vi "Create Precise Ramp Int16.vi"(8 "error in (no error)":errorcluster, 10 "Waveform":T1={"Start"=1.0, "End"=256.0, "Time"=1.0} {"Start" min=0.0 max=1.0 format="%.2f"; "Time" min=0.0 max=1.0 format="%.2f"}) -> (0 "error out":errorcluster, 2 "Waveform Data":dbl[](array[numeric]))   [LabVIEW 2013]
uses:
  PreciseRampWaveform.ctl
  <vilib>/Analysis/1siggen.llb/Ramp Pattern by Samples.vi
  <vilib>/Analysis/NI_AALBase.lvlib
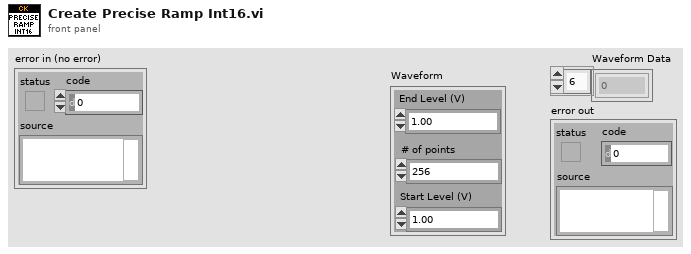
[diagram p1: front panel]
types:
  T1 = typedef "PreciseRampWaveform.ctl" = cluster{"Start":dbl, "End":dbl, "Time":dbl}
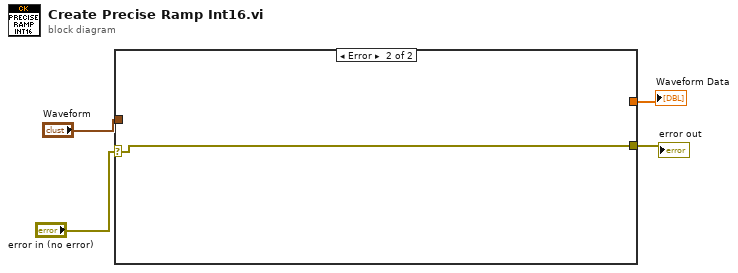
[diagram p0: block diagram]
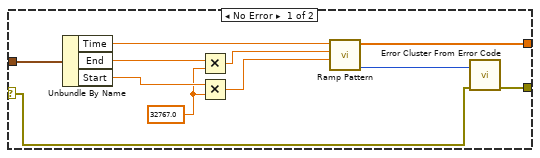
[diagram p2: hidden frame]
diagram:
  n1 = case shown="Error" "error in (no error)" {
    selector: "error in (no error)" -> [w5 w16]
    tunnel: [w14 _] -> w4
    tunnel: "Waveform" -> [w8 _]
    tunnel: [w6 w16] -> w2
    frame No Error {
      w9 = 32767.0 ("y")
      n2 = Unbundle By Name(w8) -> ("Time"=w15:dbl, "End"=w13:dbl, "Start"=w12:dbl)
      n3 = Multiply(x=w13, y=w9) -> (x*y=w11:dbl)
      n4 = Multiply(x=w12, y=w9) -> (x*y=w10:dbl)
      n5 = call-poly <vilib>:"Ramp Pattern.vi"("start"=w10, "end"=w11, "samples"=w15) -> ("error"=w7:i32, "Ramp Pattern"=w14:dbl[])  [unwired: 7 in]
      n6 = call <vilib>:"Error Cluster From Error Code.vi"("error in (no error)"=w5, "error code (0)"=w7) -> ("error out"=w6:errorcluster)  [unwired: 7 in]
    }
    frame Error {
    }
  }
  "Waveform Data" <- w4
  "error out" <- w2
